vi "ExSubOpenSpectrometer.vi"(2 "error in (no error)":errorcluster, 3 "Spectrometer Device ID":u32) -> (0 "error out":errorcluster, 1 "Spectrometer Handle":u32)   [LabVIEW 2010]
panel:
  # "ExSubOpenSpectrometer:\nThis just opens the spectrometer and nothing else."
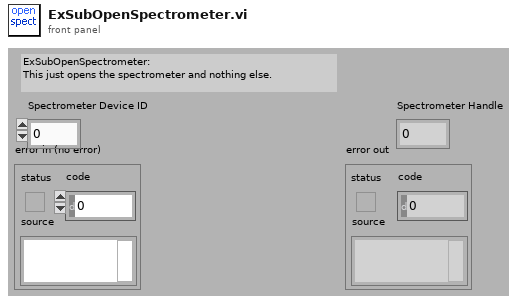
[diagram p1: front panel]
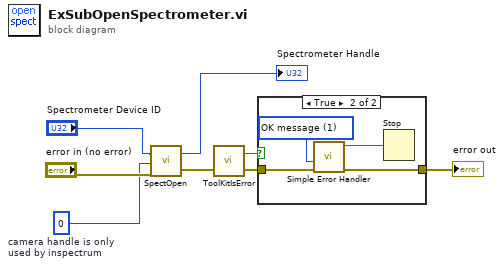
[diagram p0: block diagram]
diagram:
  w1 = 0  # camera handle is only used by inspectrum
  n1 = call <userlib>:"SpectOpen.vi"("error in"="error in (no error)", "Camera Handle"=w1, "Spectrometer ID"="Spectrometer Device ID") -> ("error out"=w8:errorcluster, "Spectrometer Handle"=→"Spectrometer Handle":u32)
  n2 = call <userlib>:"ToolKitIsError.vi"("error in"=w8) -> ("error out"=w6:errorcluster, "Error Flag"=w7:bool)  [unwired: 1 in]
  n3 = case shown="True" w7 {
    tunnel: w6 -> [w9 w13]
    tunnel: [w9 w11] -> w5
    frame False {
    }
    frame True {
      w10 = u16 1 items=["no dialog", "OK message", "continue or stop message"] ("type of dialog (OK msg:1)")
      n4 = call <vilib>:"Simple Error Handler.vi"("type of dialog (OK msg:1)"=w10, "error in (no error)"=w13) -> ("error?"=w12:bool, "error out"=w11:errorcluster)  [unwired: 3 in, 3 out]
      n5 = Stop(stop? (T)=w12) -> ()
    }
  }
  "error out" <- w5
